vi "getAllsubset.vi"(8 "error in (no error)":errorcluster, 10 "getAll":T1, 11 "instrument.PPMS3 in":refnum<class "instrument.PPMS3.lvclass">) -> (0 "error out":errorcluster, 2 "output cluster":variant, 3 "instrument.PPMS3 out":refnum<class "instrument.PPMS3.lvclass">)   [LabVIEW 2019, in "instrument.PPMS3.lvclass"]
uses:
  instrument.PPMS3.lvclass
  instrument.PPMS/Typedefs/PPMS.getAll--cluster.ctl
  instrument.PPMS/instrument.PPMS.lvclass
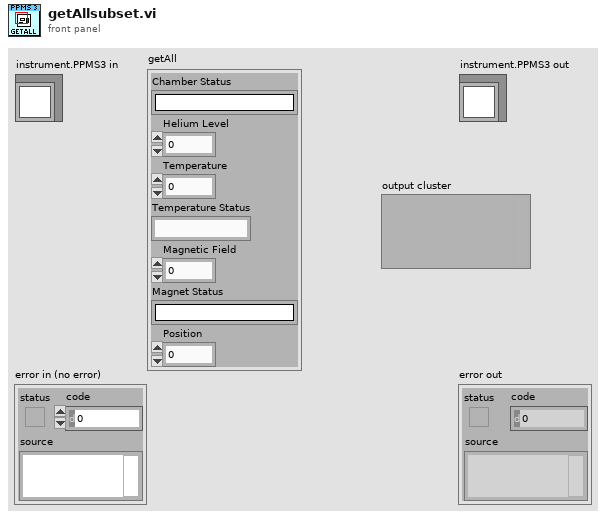
[diagram p1: front panel]
types:
  T1 = typedef "instrument.PPMS.lvclass/PPMS.getAll--cluster.ctl" = cluster{"Chamber Status":string, "Helium Level":dbl, "Temperature":dbl, "Temperature Status":string, "Magnetic Field":dbl, "Magnet Status":string, "Position":dbl}
  T2 = cluster{"Chamber Status":string, "Helium Level":dbl, "Temperature":dbl, "Temperature Status":string, "Magnetic Field":dbl, "Magnet Status":string}
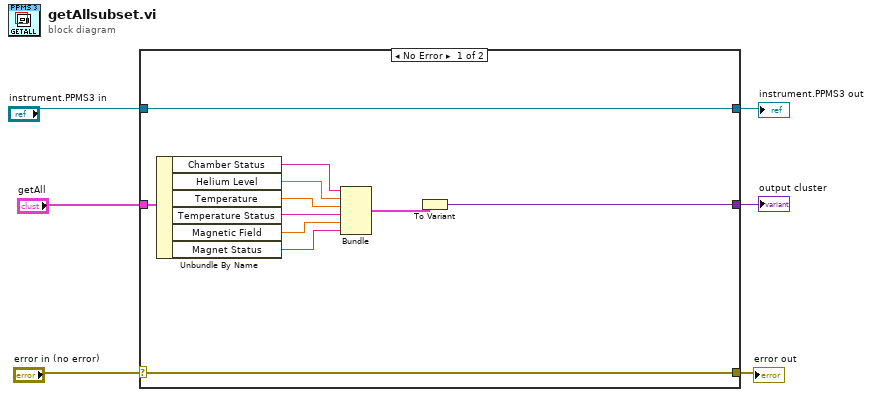
[diagram p0: block diagram]
diagram:
  n1 = case shown="No Error" "error in (no error)" {
    selector: "error in (no error)" -> [w16 w19]
    tunnel: [w16 w19] -> w6
    tunnel: [w17 w18] -> w4
    tunnel: "instrument.PPMS3 in" -> [w17 w18]
    tunnel: "getAll" -> [w8 _]
    tunnel: [w15 _] -> w5
    frame No Error {
      n2 = Unbundle By Name(w8) -> ("Chamber Status"=w9:string, "Helium Level"=w12:dbl, "Temperature"=w13:dbl, "Temperature Status"=w14:string, "Magnetic Field"=w11:dbl, "Magnet Status"=w10:string)
      n3 = Bundle("Chamber Status"=w9, "Helium Level"=w12, "Temperature"=w13, "Temperature Status"=w14, "Magnetic Field"=w11, "Magnet Status"=w10) -> (w7:T2)  [unwired: 1 in]
      n4 = To Variant(anything=w7) -> (Variant=w15:variant)
    }
    frame Error {
    }
  }
  "error out" <- w6
  "instrument.PPMS3 out" <- w4
  "output cluster" <- w5
